vi "GFITS_LibWriteFromMemeFits.vi"(8 "error in (no error)":errorcluster, 11 "imname":string) -> (0 "error out":errorcluster, 2 "return value":i32, 3 "imname out":string)   [LabVIEW 2016]
uses:
  c/lib/libgfits.so
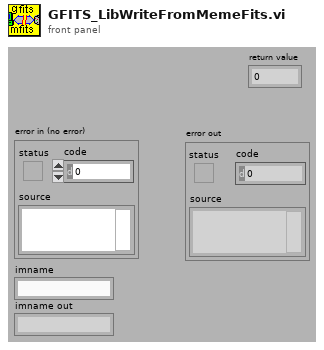
[diagram p1: front panel]
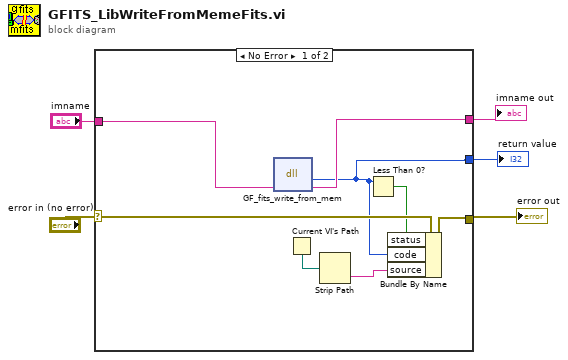
[diagram p0: block diagram]
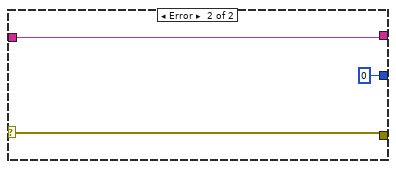
[diagram p2: hidden frame]
diagram:
  n1 = case shown="No Error" "error in (no error)" {
    selector: "error in (no error)" -> [w13 w16]
    tunnel: [w6 0] -> w5
    tunnel: [w9 w16] -> w3
    tunnel: "imname" -> [w8 w14]
    tunnel: [w7 w14] -> w1
    frame No Error {
      n2 = dll-call lib="home/simager/panview/PAN/Modules/GFITS/private/c/lib/libgfits.so" fn="GF_fits_write_from_mem"("imname"=w8) -> ("return type"=w6:i32, "imname"=w7:string)  [unwired: 3 in, 2 out]
      n3 = Current VI's Path() -> (path=w11:path)
      n4 = Strip Path(path=w11) -> (name=w10:string)  [unwired: 1 out]
      n5 = Less Than 0?(x=w6) -> (x < 0?=w12:bool)
      n6 = Bundle By Name(cluster=w13, "status"=w12, "code"=w6, "source"=w10) -> (w9:errorcluster)
    }
    frame Error {
    }
  }
  "return value" <- w5
  "error out" <- w3
  "imname out" <- w1
